vi "Flag_Read.vi"(8 "error in (no error)":errorcluster) -> (0 "error out":errorcluster, 2 "Found?":bool, 3 "Flag":T1)   [LabVIEW 2016, in "SeqProcessor.lvlib"]
uses:
  SeqProcessor.lvlib
  controls/Flag.ctl
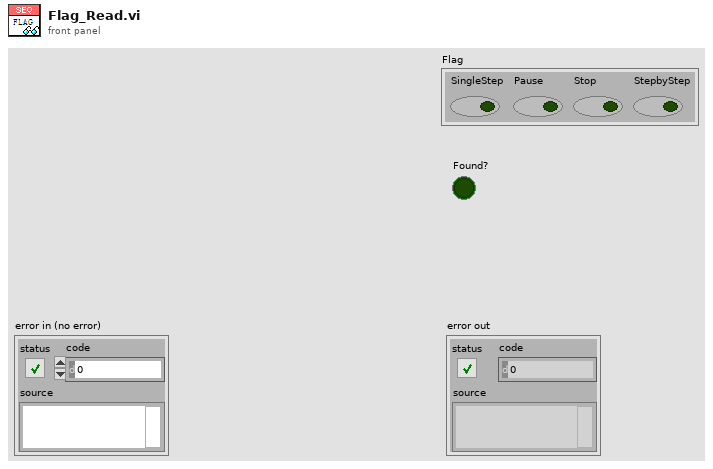
[diagram p1: front panel]
types:
  T1 = typedef "SeqProcessor.lvlib/Flag.ctl" = cluster{"SingleStep":bool, "Pause":bool, "Stop":bool, "StepbyStep":bool}
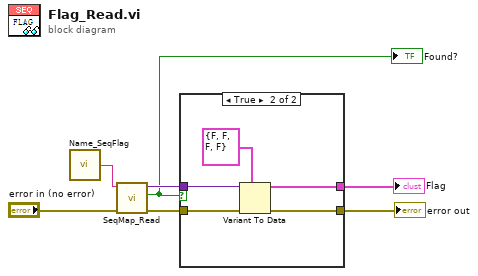
[diagram p0: block diagram]
diagram:
  n1 = call "Name_SeqFlag.vi"() -> ("SeqFlag"=w4:string)  [unwired: 5 in]
  n2 = call "SeqMap_Read.vi"("error in (no error)"="error in (no error)", "Tag"=w4) -> ("Error Out"=w3:errorcluster, "Found?"=w1:bool, "Value"=w2:variant)  [unwired: 7 in]
  "Found?" <- w1
  n3 = case shown="True" w1 {
    tunnel: w3 -> [w8 w13]
    tunnel: [w8 w12] -> w7
    tunnel: w2 -> [_ w11]
    tunnel: [_ w10] -> w6
    frame False {
    }
    frame True {
      n4 = Variant To Data(error in=w13, type=T1 {"SingleStep"=FALSE, "Pause"=FALSE, "Stop"=FALSE, "StepbyStep"=FALSE} ("Flag"), Variant=w11) -> (data=w10:T1, error out=w12:errorcluster)
    }
  }
  "error out" <- w7
  "Flag" <- w6
